vi "Get Technology.vi"(8 "error in (no error)":errorcluster, 11 "niDTS WLAN Dut in":refnum<class "niDTS WLAN Dut.lvclass">) -> (0 "error out":errorcluster, 2 "Technolgy":T1="WLAN", 3 "niDTS WLAN Dut out":refnum<class "niDTS WLAN Dut.lvclass">)   [LabVIEW 2015, in "niDTS WLAN.lvlib" / "niDTS WLAN Dut.lvclass"]
uses:
  niDTS WLAN Dut.lvclass
  Framework/Test/Includes/niDTS Test INC Technology.ctl
  Framework/niDTS Framework.lvlib
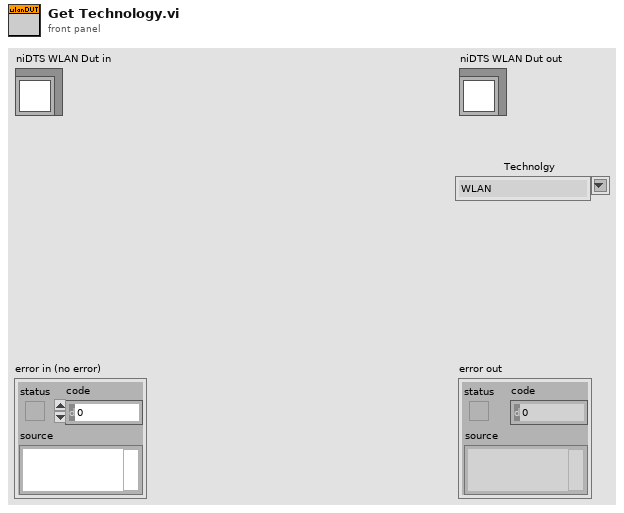
[diagram p1: front panel]
types:
  T1 = typedef "niDTS Framework.lvlib/niDTS Test INC Technology.ctl" = string
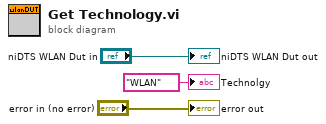
[diagram p0: block diagram]
diagram:
  "error out" <- "error in (no error)"
  "niDTS WLAN Dut out" <- "niDTS WLAN Dut in"
  "Technolgy" <- T1 "WLAN" ("Technolgy")
